vi "Get Response Timeout.vi"(0 "LVx In":refnum<class "LVx.lvclass">, 11 "error in (no error)":errorcluster) -> (4 "LVx Out":refnum<class "LVx.lvclass">, 8 "timeout in ms (-1:never)":i32=-1, 15 "error out":errorcluster)   [LabVIEW 2011, in "LVx.lvlib" / "LVx.lvclass"]
uses:
  LVx.lvclass
  LVx.lvclass/LVx.ctl
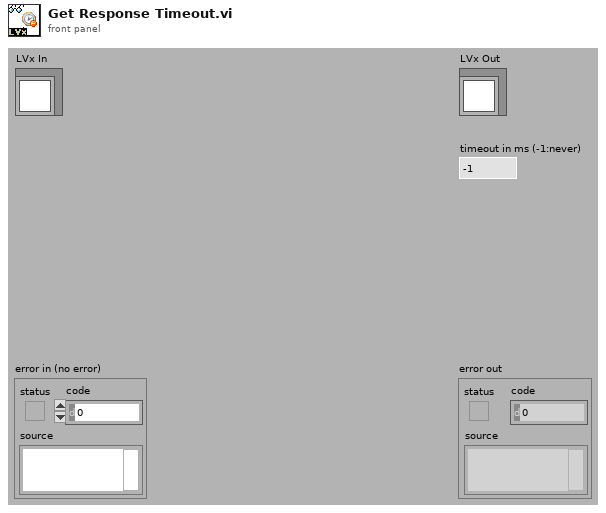
[diagram p1: front panel]
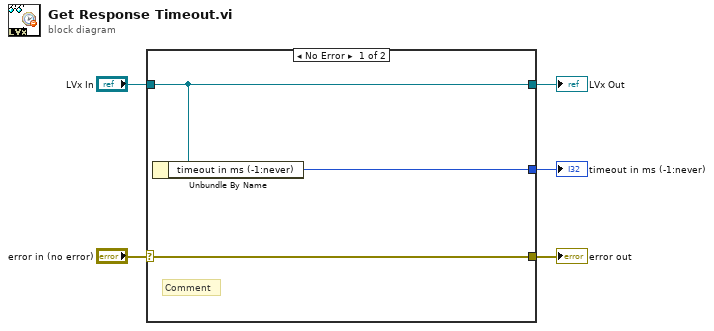
[diagram p0: block diagram]
diagram:
  n1 = case shown="No Error" "error in (no error)" {
    selector: "error in (no error)" -> [w8 w9]
    tunnel: [w8 w9] -> w4
    tunnel: [w7 w10] -> w2
    tunnel: "LVx In" -> [w7 w10]
    tunnel: [w6 _] -> w1
    frame No Error {
      # "Comment"
      n2 = Unbundle By Name(w7) -> ("timeout in ms (-1:never)"=w6:i32)
    }
    frame Error {
    }
  }
  "error out" <- w4
  "LVx Out" <- w2
  "timeout in ms (-1:never)" <- w1
